vi "Modbus.WriteMultipleCoils.vi"(8 "error in (no error)":errorcluster, 11 "address":T1) -> (0 "error out":errorcluster)   [LabVIEW 2019, in "Modbus.lvlib"]
uses:
  Modbus.lvlib
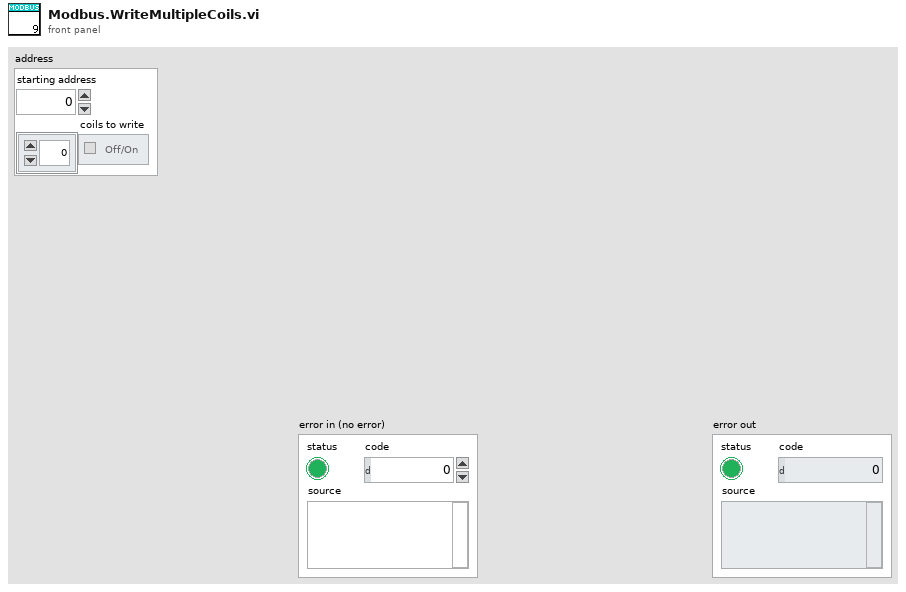
[diagram p1: front panel]
types:
  T1 = cluster{"starting address":u16, "coils to write":bool[]}
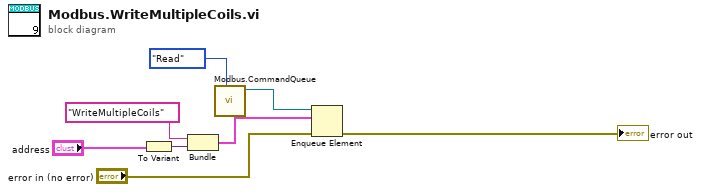
[diagram p0: block diagram]
diagram:
  n1 = To Variant(anything="address") -> (Variant=w4:variant)
  n2 = Bundle("WriteMultipleCoils", "Variant"=w4) -> (w5:cluster{string, "Variant":variant})  [unwired: 1 in]
  n3 = call "Modbus.CommandQueue.vi"("OP"=enum16{"Read", "Write"}."Read") -> ("queue OUT"=w7:refnum<queue>)  [unwired: 10 in]
  n4 = Enqueue Element(queue=w7, element=w5, error in (no error)="error in (no error)") -> (error out=→"error out":errorcluster)  [unwired: 1 in, 2 out]
